vi "sub_SDR_rx_ApplyMatchedFilter.vi"(7 "Filter Options":T1={"Samples per symbol"=2, "Roll-Off"=1.0, "Filter length (symbols)"=4}, 10 "Received stream":cdb[](array[numeric])) -> (2 "Received Symbols":cdb[](array[numeric]))   [LabVIEW 2012]
uses:
  <vilib>/Analysis/2dsp.llb/1D Convolution (CDB).vi
  <vilib>/Analysis/2dsp.llb/Decimate (single shot, CDB).vi
  <vilib>/Analysis/NI_AALPro.lvlib
  <vilib>/addons/Modulation/niDMT.lvlib
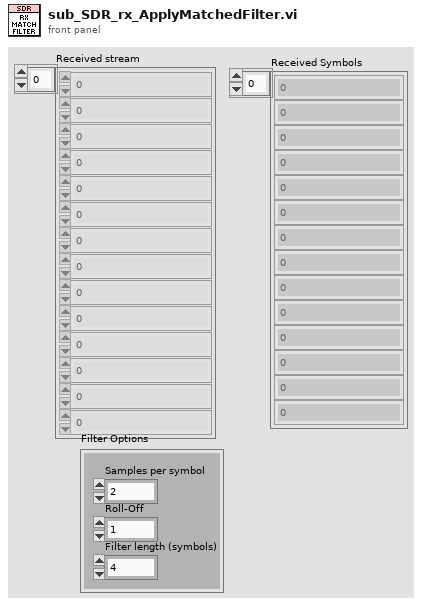
[diagram p1: front panel]
types:
  T1 = cluster{"Samples per symbol":i32, "Roll-Off":dbl, "Filter length (symbols)":i32}
  T2 = enum16{"FSK", "PSK", "QAM", "MSK", "PAM", "ASK", "CPM"}
  T3 = enum16{"none", "Raised Cosine", "Root Raised Cos", "Gaussian"}
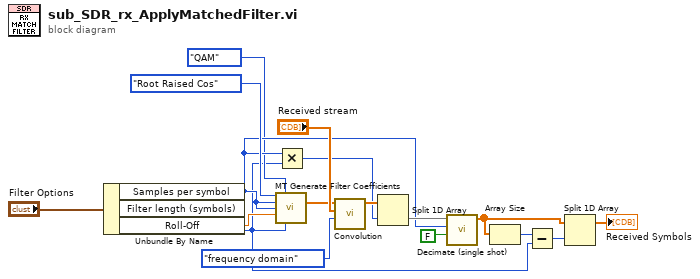
[diagram p0: block diagram]
diagram:
  n1 = Unbundle By Name("Filter Options") -> ("Samples per symbol"=w7:i32, "Filter length (symbols)"=w1:i32, "Roll-Off"=w6:dbl)
  n2 = call <vilib>:"MT Generate Filter Coefficients.vi"("pulse shaping filter (none)"=T3."Root Raised Cos", "modulation type"=T2."QAM", "pulse shaping samples per symbol (16)"=w7, "matched samples per symbol (16)"=w7, "filter parameter"=w6, "filter length (symbols)"=w1) -> ("matched filter coefficients"=w4:dbl[])  [unwired: 7 in, 2 out]
  n3 = Multiply(x=w7, y=w1) -> (x*y=w3:i32)
  n4 = call-poly <vilib>:"Convolution.vi"("algorithm"=enum32{"direct", "frequency domain"}."frequency domain", "Y"="Received stream", "X"=w4) -> ("X * Y"=w13:cdb[])  [unwired: 7 in, 1 out]
  n5 = Split 1D Array(array=w13, index=w3) -> (second subarray=w16:cdb[])  [unwired: 1 out]
  n6 = call-poly <vilib>:"Decimate (single shot).vi"("averaging"=FALSE, "decimating factor"=w7, "X"=w16) -> ("Decimated Array"=w10:cdb[])  [unwired: 7 in, 1 out]
  n7 = Array Size(array=w10) -> (size(s)=w12:i32)
  n8 = Subtract(x=w12, y=w1) -> (x-y=w11:i32)
  n9 = Split 1D Array(array=w10, index=w11) -> (first subarray=→"Received Symbols":cdb[])  [unwired: 1 out]
